vi "Periodic Tasks.vi"(8 "error in":errorcluster) -> ()   [LabVIEW 2011]
doc: "This VI runs in parallel to other tasks. It can contain as many user-defined periodic loops as you need. These can carry out PID or other sorts of timed response."
uses:
  <vilib>/Rock Robotics/WPI/DriverStation/WPI_DriverStationRobotMode.ctl
  <vilib>/Rock Robotics/SystemInterfaces/Utilities/FPGA_UtilitiesLED State.ctl
  <vilib>/Rock Robotics/SystemInterfaces/Utilities/FPGA_UtilitiesLED Source.ctl
  Robot Global Data.vi
  <vilib>/Rock Robotics/WPI/Solenoid/Deprecated/WPI_SolenoidSetBool.vi
  <vilib>/Rock Robotics/WPI/Compressor/WPI_CompressorGetSetRefNum.vi
  <vilib>/addons/control/pid/NI_PID_pid.lvlib
  <vilib>/addons/control/pid/pid.llb/PID (DBL).vi
panel:
  out "Turret Joystick":dbl(slide) scale=-1.0..1.0
  out "PID Output":dbl(slide) scale=-1.0..1.0
  out "Target Pot":dbl(slide) scale=2.0..3.5
  in  "Min Turret Output":dbl
  # "!!!DISABLED!!!"
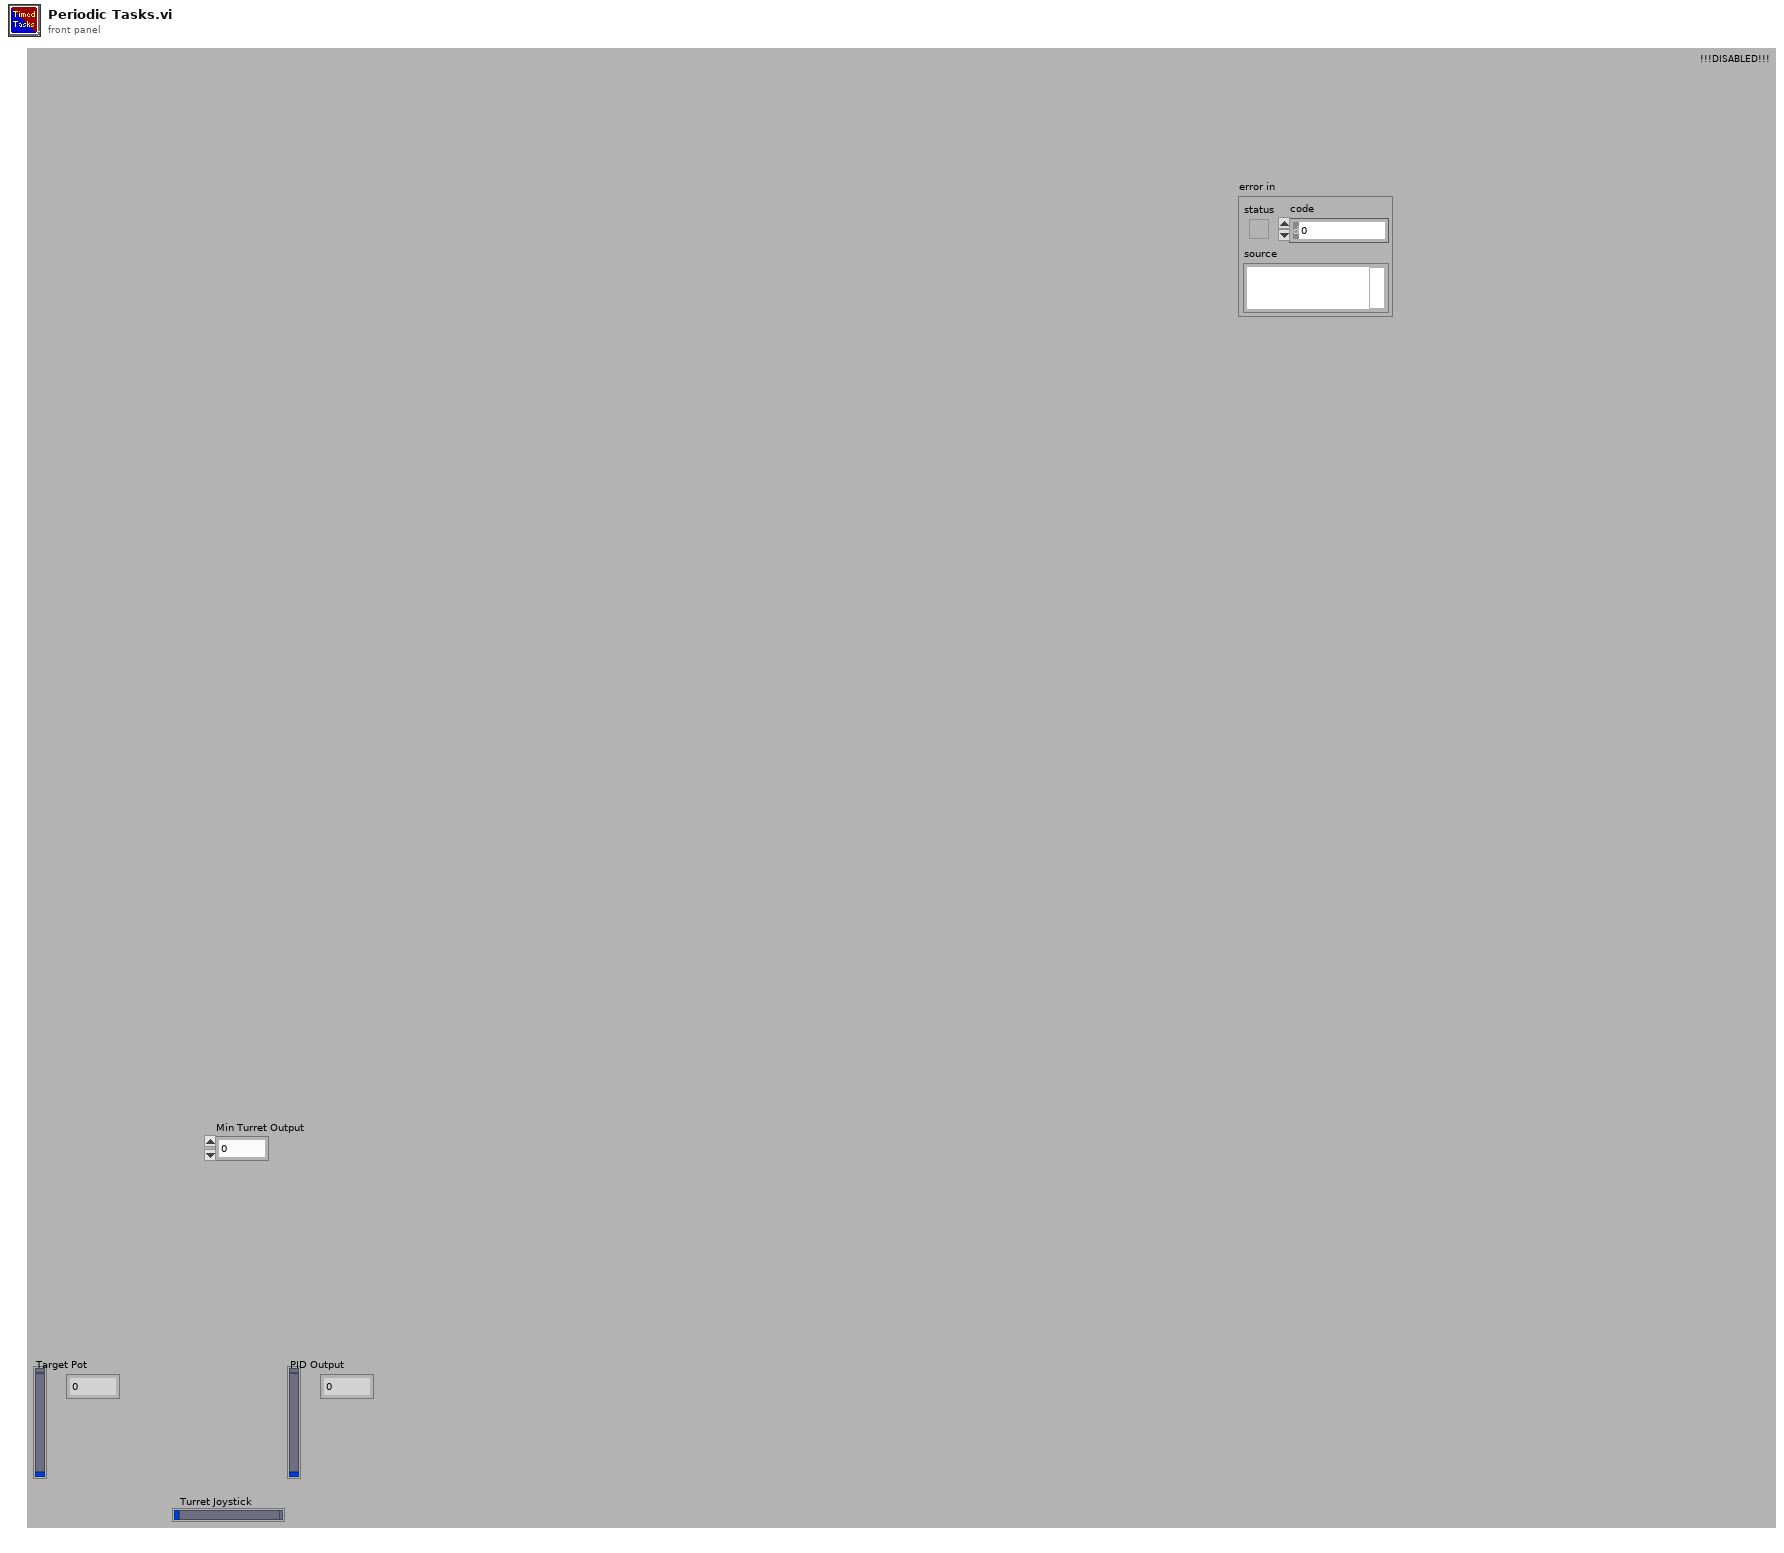
[diagram p1: front panel]
types:
  T1 = typedef "WPI_DriverStationRobotMode.ctl" = enum16{"Autonomous Disabled", "Autonomous Enabled", "Teleop Disabled", "Teleop Enabled", "Timeout", "Finish"}
  T2 = cluster{"proportional gain (Kc)":dbl, "integral time (Ti, min)":dbl, "derivative time (Td, min)":dbl}
  T3 = typedef "WPI_AnalogChannelDevRef.ctl" = cluster{"DevStatus":errorcluster, "Analog Module":T4, "Analog Channel":T5}
  T4 = typedef "FPGA_TypedefAnalogModule.ctl" = enum16{"Analog Module 1", "Analog Module 2"}
  T5 = typedef "FPGA_AIChannel.ctl" = enum8{"AI 1", "AI 2", "AI 3", "AI 4", "AI 5", "AI 6", "AI 7", "AI 8", "Invalid"}
  T6 = typedef "WPI_MotorControlDeviceRef.ctl" = cluster{"DeviceStatus":errorcluster, "Type":enum16{"PWM", "CAN"}, "PWM":cluster{"Digital Module":T7, "PWM Channel":T8, "DeadBand":T9}, "CAN":cluster{"Device Number":u8, "Control Mode":T10, "Semaphore":T11, "Max Vout":dbl}, "Invert":bool, "TransformRef":T12, "InvTransformRef":T12}
  T7 = typedef "FPGA_TypedefDigitalModule.ctl" = enum16{"Digital Module 1", "Digital Module 2"}
  T8 = typedef "FPGA_DIOPWMChannel.ctl" = enum8{"PWM 1", "PWM 2", "PWM 3", "PWM 4", "PWM 5", "PWM 6", "PWM 7", "PWM 8", "PWM 9", "PWM 10", "Invalid"}
  T9 = typedef "WPI_PWMDeadband.ctl" = cluster{"Name":string, "maxPositivePwm":i32, "minPositivePwm":i32, "centerPwm":i32, "maxNegativePwm":i32, "minNegativePwm":i32, "angularRange":u16}
  T10 = typedef "WPI_CANJaguar_ControlMode.ctl" = enum8{"Percent VBus", "Current", "Speed", "Position", "Voltage"}
  T11 = typedef "Semaphore RefNum" = refnum<k1>
  T12 = typedef "WPI_PWMTransform_ConPane.ctl" = refnum<vi>
  T13 = cluster{"axis 1 (x)":dbl, "axis 2 (y)":dbl, "axis 3 (throttle)":dbl, "axis 4":dbl, "axis 5":dbl, "axis 6":dbl}
  T14 = typedef "WPI_JoystickButtonState.ctl" = cluster{"Button 1":bool, "Button 2":bool, "Button 3":bool, "Button 4":bool, "Button 5":bool, "Button 6":bool, "Button 7":bool, "Button 8":bool, "Button 9":bool, "Button 10":bool, "Button 11":bool, "Button 12":bool}
  T15 = typedef "UDP Dashboard Packet TypeDef.ctl" = cluster{"Distance":dbl, "Shooter Control":cluster{"Manual Enabled":bool, "Manual Distance":dbl, "Power Constant":dbl, "RPM Constant":dbl, "Layup Distance":dbl, "RPM Range":cluster{"Max Percentage":dbl, "Min Percentage":dbl}, "Dt In":dbl}, "Tracking Setpoint":dbl, "Shooter PID gains":cluster{"proportional gain (Kc)":dbl, "integral time (Ti, min)":dbl, "derivative time (Td, min)":dbl}, "Tracking PID gains":cluster{"proportional gain (Kc)":dbl, "integral time (Ti, min)":dbl, "derivative time (Td, min)":dbl}, "Shooter PID gains 2":cluster{"proportional gain (Kc)":dbl, "integral time (Ti, min)":dbl, "derivative time (Td, min)":dbl}, "Tracking Tolerance":dbl, "Tracking Limit":dbl, "Autonomous Ball Collection / Shoot Period":dbl}
  T16 = cluster{"Target Pot":dbl, "Motor Output":dbl, "Current Voltage":dbl}
  T17 = typedef "WPI_CompressorDevRef.ctl" = cluster{"DevStatus":errorcluster, "DigitalInputDevRef":T18, "RelayDevRef":T20}
  T18 = typedef "WPI_DigitalInputDevRef.ctl" = cluster{"DevStatus":errorcluster, "DIO Channel":T19, "Digital Module":T7}
  T19 = typedef "FPGA_DIOChannel.ctl" = enum8{"DIO 1", "DIO 2", "DIO 3", "DIO 4", "DIO 5", "DIO 6", "DIO 7", "DIO 8", "DIO 9", "DIO 10", "DIO 11", "DIO 12", "DIO 13", "DIO 14", "Invalid"}
  T20 = typedef "WPI_RelayDevRef.ctl" = cluster{"DevStatus":errorcluster, "Relay Channel":T21, "Digital Module":T7, "Relay Direction":T22}
  T21 = typedef "FPGA_DIORelayChannel.ctl" = enum8{"Relay 1", "Relay 2", "Relay 3", "Relay 4", "Relay 5", "Relay 6", "Relay 7", "Relay 8", "Invalid"}
  T22 = typedef "WPI_RelayDirection.ctl" = enum16{"Both directions", "Forward only", "Reverse only"}
  T23 = typedef "WPI_SolenoidDevRef.ctl" = cluster{"DevStatus":errorcluster, "Solenoid Module":T24, "Forward Solenoid Channel":T25, "Reverse Solenoid Channel":T25}
  T24 = typedef "FPGA_TypedefSolenoidModule.ctl" = enum16{"Solenoid Module 1", "Solenoid Module 2"}
  T25 = typedef "WPI_SolenoidChannel.ctl" = enum8{"Solenoid 1", "Solenoid 2", "Solenoid 3", "Solenoid 4", "Solenoid 5", "Solenoid 6", "Solenoid 7", "Solenoid 8", "Invalid"}
  T26 = typedef "WPI_GyroDevRef.ctl" = cluster{"DevStatus":errorcluster, "Analog Module":T4, "Analog Channel":T5, "Offset":dbl, "Gain (VoltsPerDegree/Second)":dbl}
  T27 = cluster{"Gear Shifter":bool, "Tipper":bool, "Tipper Lock":bool, "Stabilizer":bool}
  T28 = cluster{"Shooter Warmup":bool, "Shooter Allow Fire":bool}
  T29 = cluster{"Front Roller":bool, "Back Roller":bool, "Lower Mag":bool, "Upper Mag":bool, "Front Enter":bool, "Rear Enter":bool}
  T30 = cluster{"Current State":u32, "Reading State":u32, "Number of Balls":u32, "State":enum16{"Load Balls", "Shoot", "Wait"}}
  T31 = typedef "FPGA_UtilitiesLED State.ctl" = enum16{"Off", "On", "Toggle"}
  T32 = typedef "FPGA_UtilitiesLED Source.ctl" = enum16{"User LED", "FPGA LED"}
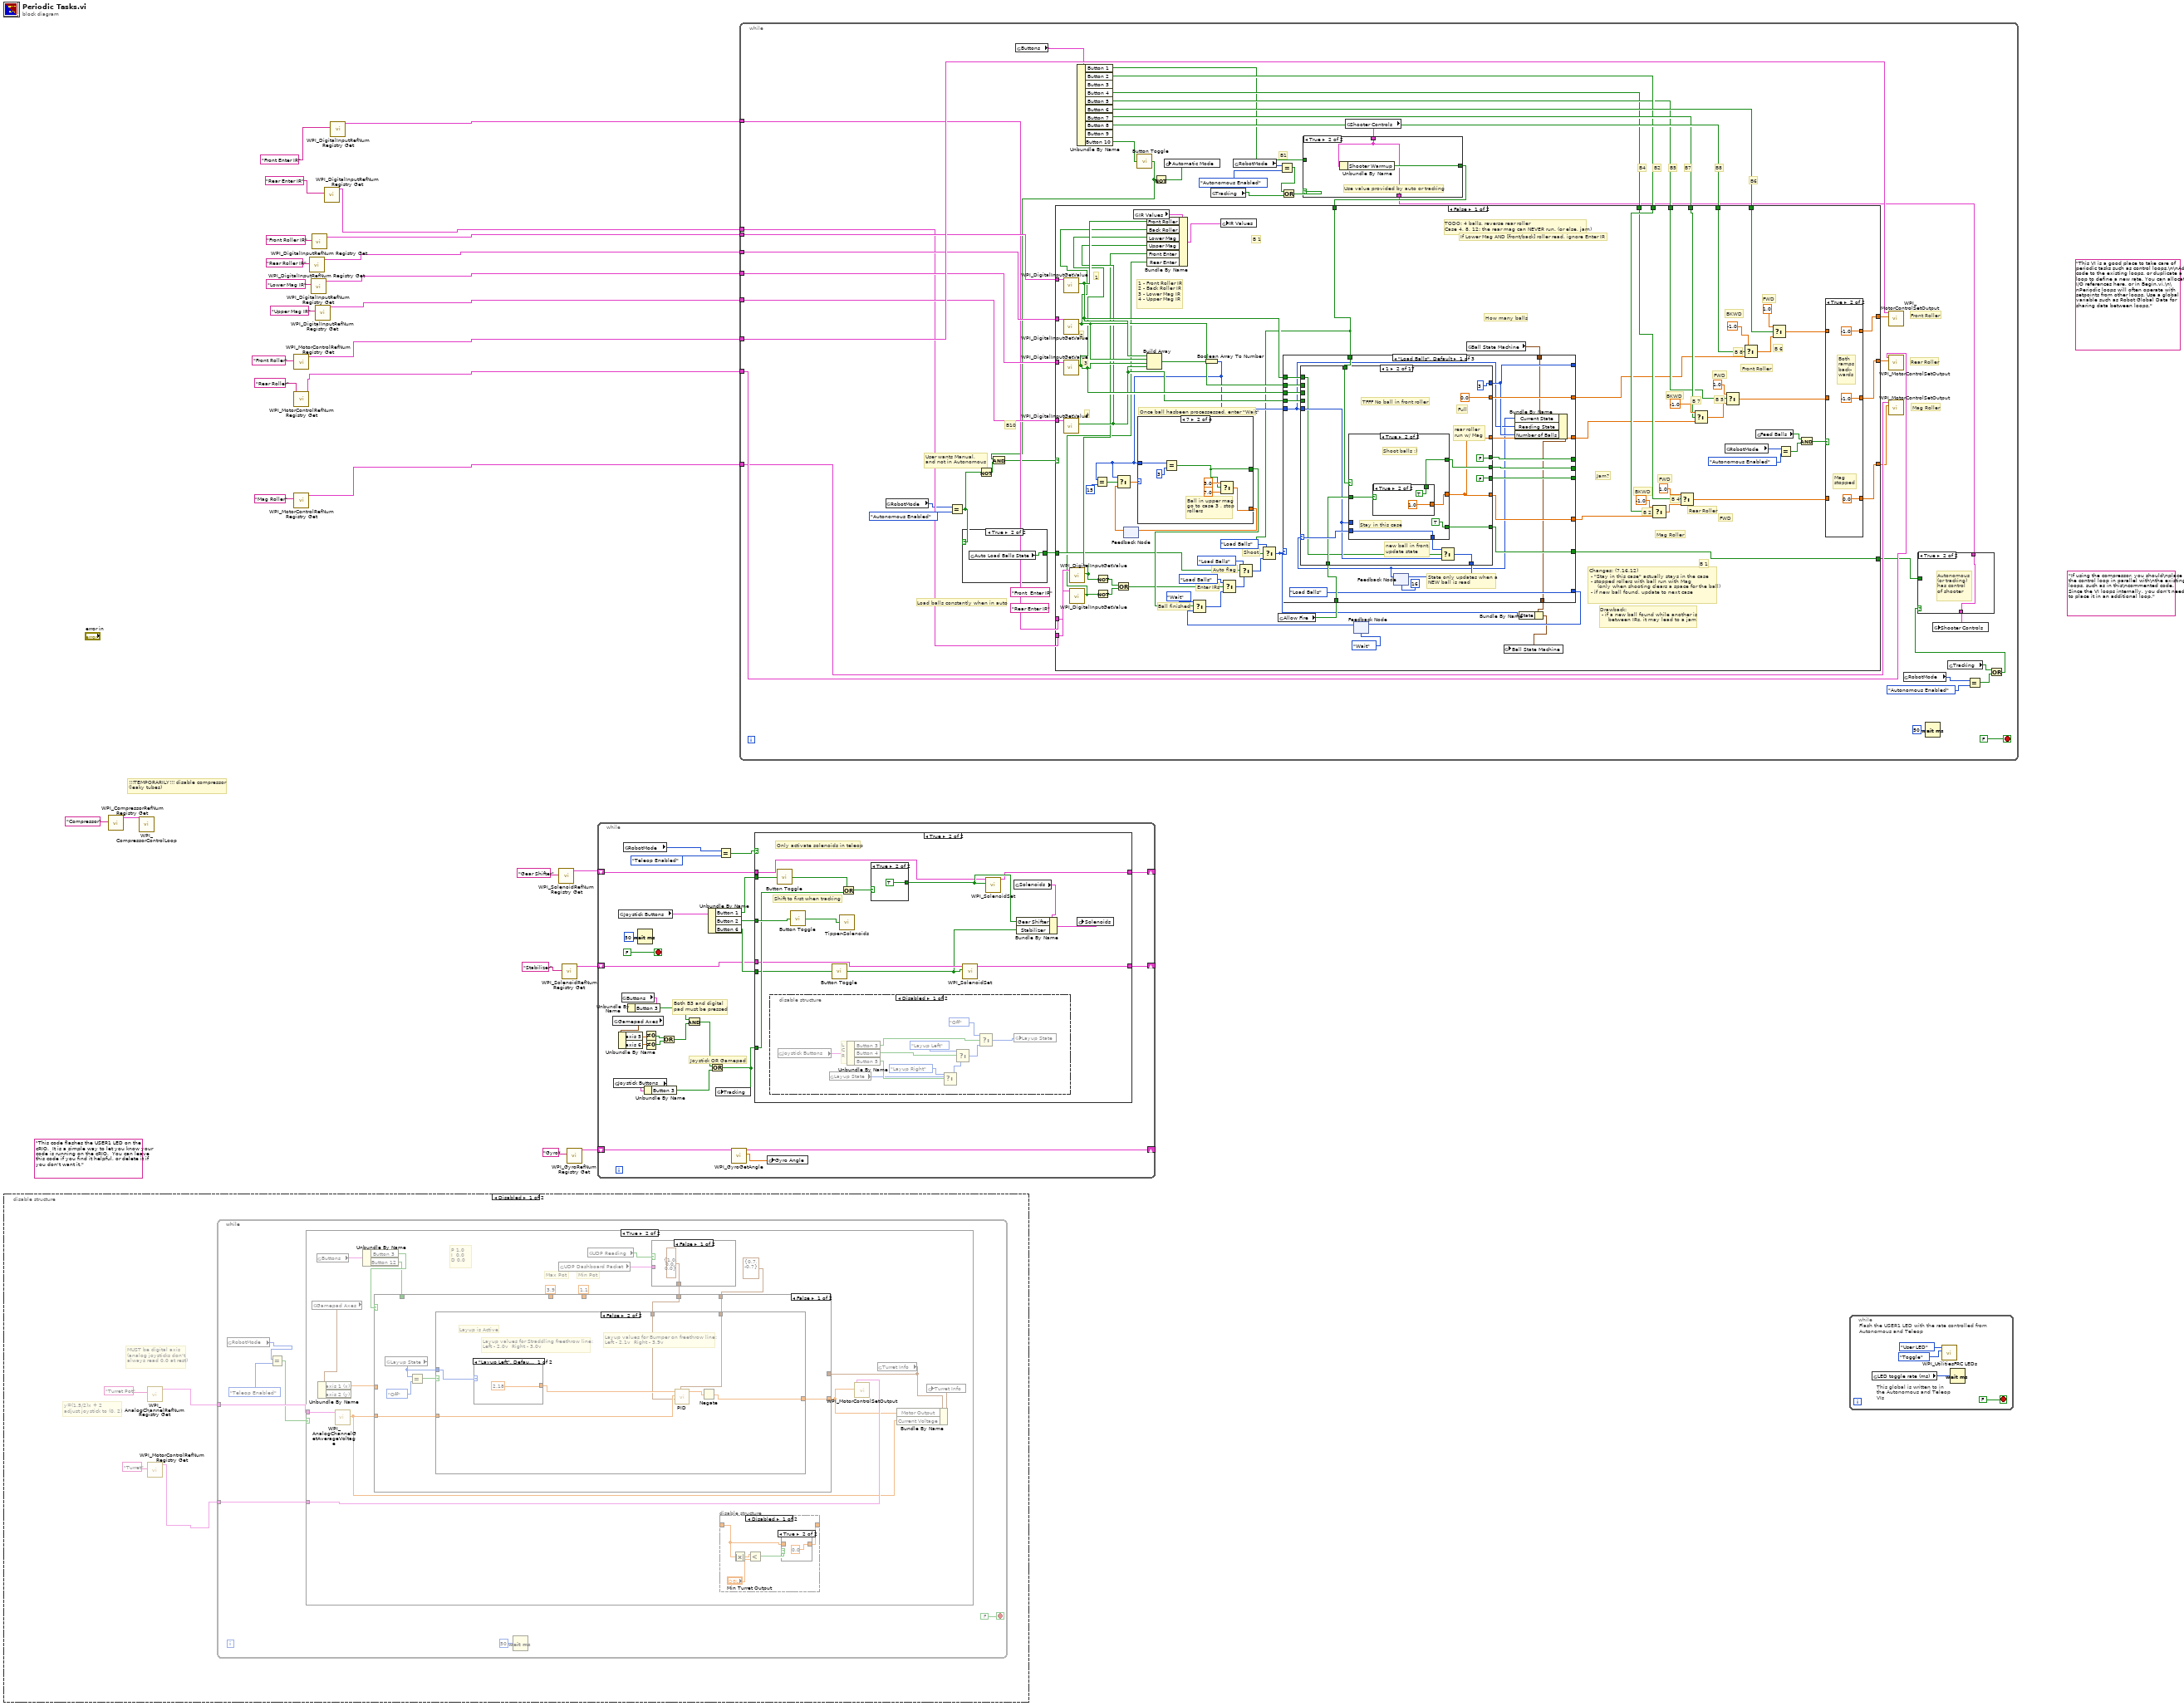
[diagram p0: block diagram]
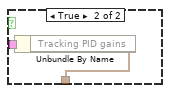
[diagram p3: hidden frame]
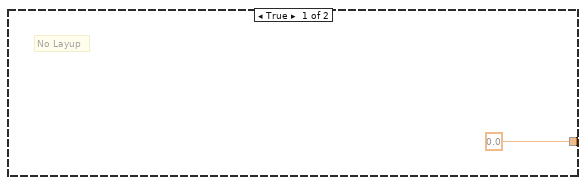
[diagram p4: hidden frame]
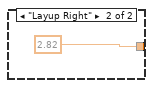
[diagram p5: hidden frame]
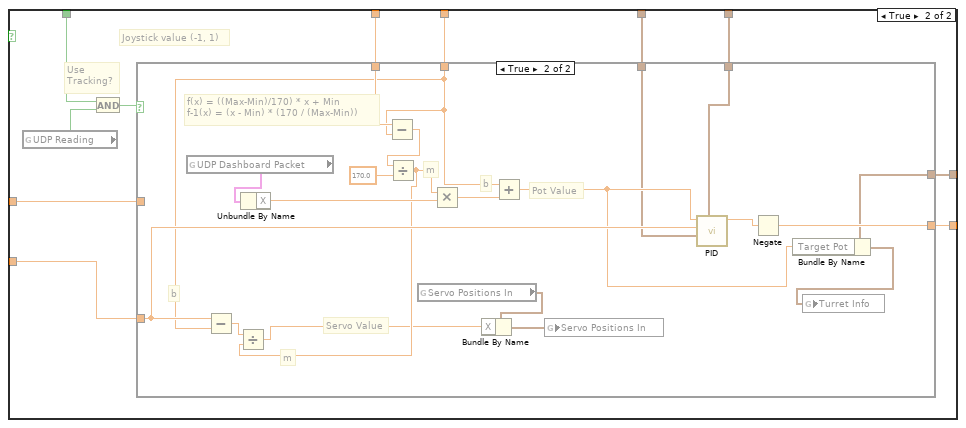
[diagram p6: hidden frame]
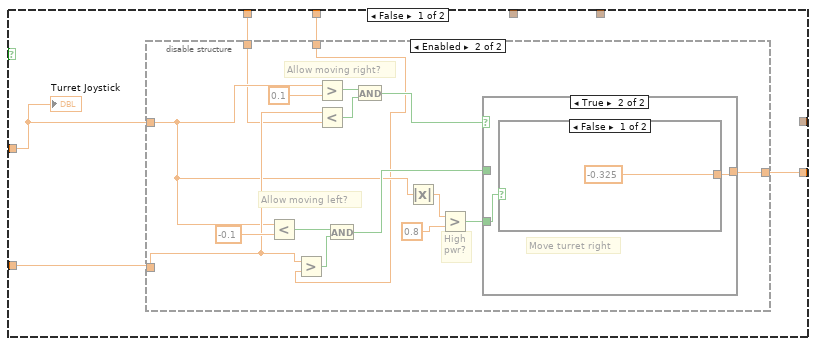
[diagram p7: hidden frame]
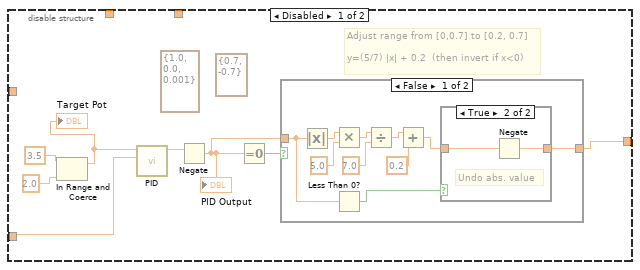
[diagram p8: hidden frame]
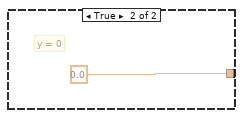
[diagram p10: hidden frame]
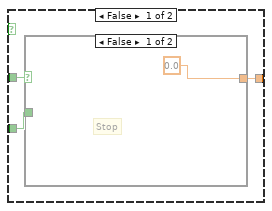
[diagram p11: hidden frame]
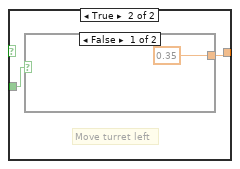
[diagram p12: hidden frame]
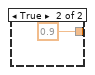
[diagram p13: hidden frame]
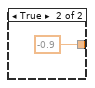
[diagram p14: hidden frame]
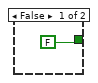
[diagram p20: hidden frame]
diagram:
  (unwired) "If using the compressor, you should\nplace the control loop in parallel with\nthe existing loops, such as in this\ncommented code. Since the VI loops internally, you don't need to place it in an additional loop."
  (unwired) "This code flashes the USER1 LED on the cRIO.  It is a simple way to let you know your code is running on the cRIO.  You can leave this code if you find it helpful, or delete it if you don't want it."
  (unwired) "This VI is a good place to take care of periodic tasks such as control loops.\n\nAdd code to the existing loops, or duplicate a loop to define a new rate. You can allocate I/O references here, or in Begin.vi.\n\nPeriodic loops will often operate with setpoints from other loops. Use a global variable such as Robot Global Data for sharing data between loops."
  # "!!!TEMPORARILY!!! disable compressor\n(leaky tubes)"
  n1 = disable-structure shown="Disabled" {
    frame Disabled {
      # "MUST be digital axis\n(analog joysticks don't\nalways read 0.0 at rest)"
      # "y=(1.5/2)x + 2\nadjust joystick to (0, 2)"
      n2 = call <vilib>:"WPI_AnalogChannelRefNum Registry Get.vi"("refnum name"="Turret Pot") -> ("AIDeviceRef"=w28:T3)  [unwired: 9 in, 1 out]
      n3 = call <vilib>:"WPI_MotorControlRefNum Registry Get.vi"("refnum name"="Turret") -> ("MotorControlDevRef"=w27:T6)  [unwired: 9 in, 1 out]
      n4 = while {
        tunnel: w27 -> [w36]
        tunnel: w28 -> [w34]
        stop <- FALSE stop-if-true
        n5 = global read "Robot Global Data.vi" "RobotMode"() -> (w33:T1)
        n6 = Equal?(x=w33, y=WPI_DriverStationRobotMode."Teleop Enabled" ("Robot Mode")) -> (x = y?=w31:bool)
        n7 = case shown="True" w31 {
          tunnel: w36 -> [_ w50]
          tunnel: w34 -> [_ w42]
          frame False {
          }
          frame True {
            # "Min Pot"
            # "Max Pot"
            # "P 1.0\nI  0.0\nD 0.0"
            n8 = global read "Robot Global Data.vi" "Gamepad Axes"() -> (w53:T13)
            n9 = global read "Robot Global Data.vi" "Buttons"() -> (w54:T14)
            n10 = Unbundle By Name(w53) -> ("axis 1 (x)"=w52:dbl)  [unwired: 1 out]
            n11 = call <vilib>:"WPI_AnalogChannelGetAverageVoltage.vi"("AIDeviceRef"=w42) -> ("Voltage"=w44:dbl)  [unwired: 8 in, 2 out]
            n12 = Unbundle By Name(w54) -> ("Button 3"=w51:bool, "Button 12"=w49:bool)
            n13 = global read "Robot Global Data.vi" "UDP Dashboard Packet"() -> (w39:T15)
            n14 = global read "Robot Global Data.vi" "UDP Reading"() -> (w40:bool)
            n15 = case shown="False" w40 {
              tunnel: [T2 {"proportional gain (Kc)"=1.0, "integral time (Ti, min)"=0.0, "derivative time (Td, min)"=0.0} ("PID gains") w56] -> w41
              tunnel: w39 -> [_ w57]
              frame False {
              }
              frame True {
                n16 = Unbundle By Name(w57) -> ("Tracking PID gains"=w56:T2)
              }
            }
            n17 = disable-structure shown="Disabled" {
              disable-tunnel: _ -> [w162 _]
              disable-tunnel: [w161 _] -> _
              frame Disabled {
                n18 = Absolute Value(x=w162) -> (abs(x)=w165:dbl)
                n19 = Less?(x=w165, y="Min Turret Output") -> (x < y?=w163:bool)
                n20 = case shown="True" w163 {
                  tunnel: [w166 0.0] -> w161
                  tunnel: w162 -> [w166 _]
                  frame False {
                  }
                  frame True {
                  }
                }
              }
              frame Enabled {
              }
            }
            n21 = global read "Robot Global Data.vi" "Turret Info"() -> (w43:T16)
            n22 = case shown="False" w51 {
              tunnel: w52 -> [_ w83]
              tunnel: w44 -> [w63 w85]
              tunnel: [w64 w84] -> w45
              tunnel: w49 -> [_ w81]
              tunnel: 3.9 ("y") -> [_ w79]
              tunnel: 1.1 ("y") -> [_ w78]
              tunnel: w43 -> [_ w77]
              tunnel: w41 -> [w58 w76]
              tunnel: cluster{"output high":dbl, "output low":dbl} {"output high"=0.7, "output low"=-0.7} ("output range") -> [w59 w75]
              frame False {
                n23 = global read "Robot Global Data.vi" "Layup State"() -> (w60:enum16{"Layup Left", "Layup Right", "Off"})
                n24 = Equal?(x=w60, y=enum16{"Layup Left", "Layup Right", "Off"}."Off") -> (x = y?=w62:bool)
                n25 = case shown="False" w62 {
                  tunnel: [0.0 w71] -> w64
                  tunnel: w63 -> [_ w70]
                  tunnel: w60 -> [_ w69]
                  tunnel: w59 -> [_ w67]
                  tunnel: w58 -> [_ w66]
                  frame True {
                    # "No Layup"
                  }
                  frame False {
                    # "Layup values for Bumper on freethrow line:\nLeft - 2.1v  Right - 3.9v"
                    # "Layup values for Straddling freethrow line:\nLeft - 2.0v  Right - 3.0v"
                    # "Layup is Active"
                    n26 = case shown="\"Layup Left\", Default" w69 {
                      tunnel: [2.18 ("y") 2.82 ("y")] -> w68
                      frame "Layup Left", Default {
                      }
                      frame "Layup Right" {
                      }
                    }
                    n27 = call-poly <vilib>:"PID.vi"("output range"=w67, "PID gains"=w66, "process variable"=w70, "setpoint"=w68) -> ("output"=w72:dbl)  [unwired: 6 in, 1 out]
                    n28 = Negate(x=w72) -> (-x=w71:dbl)
                  }
                }
              }
              frame True {
                # "Use \nTracking?"
                # "Joystick value (-1, 1)"
                n29 = global read "Robot Global Data.vi" "UDP Reading"() -> (w82:bool)
                n30 = And(x=w81, y=w82) -> (x .and. y?=w80:bool)
                n31 = case shown="True" w80 {
                  tunnel: w85 -> [w90 w148]
                  tunnel: [w89 w154] -> w84
                  tunnel: w83 -> [w88 _]
                  tunnel: w79 -> [w87 w159]
                  tunnel: w78 -> [w86 w147]
                  tunnel: w77 -> [_ w151]
                  tunnel: w76 -> [_ w142]
                  tunnel: w75 -> [_ w141]
                  frame False {
                    n32 = disable-structure shown="Enabled" {
                      disable-tunnel: w90 -> [w96 w119]
                      disable-tunnel: [w91 w128] -> w89
                      disable-tunnel: w88 -> [_ w116]
                      disable-tunnel: w87 -> [_ w114]
                      disable-tunnel: w86 -> [_ w113]
                      frame Disabled {
                        (unwired) T2 {"proportional gain (Kc)"=1.0, "integral time (Ti, min)"=0.0, "derivative time (Td, min)"=0.001} ("PID gains")
                        (unwired) cluster{"output high":dbl, "output low":dbl} {"output high"=0.7, "output low"=-0.7} ("output range")
                        # "Adjust range from [0,0.7] to [0.2, 0.7]\n\ny=(5/7) |x| + 0.2  (then invert if x<0)"
                        n33 = In Range and Coerce(upper limit=3.5, lower limit=2.0) -> (coerced(x)=w95:dbl)  [unwired: 1 in, 1 out]
                        "Target Pot" <- w95
                        n34 = call-poly <vilib>:"PID.vi"("process variable"=w96, "setpoint"=w95) -> ("output"=w94:dbl)  [unwired: 8 in, 1 out]
                        n35 = Negate(x=w94) -> (-x=w92:dbl)
                        "PID Output" <- w92
                        n36 = Equal To 0?(x=w92) -> (x = 0?=w93:bool)
                        n37 = case shown="False" w93 {
                          tunnel: w92 -> [w102 _]
                          tunnel: [w99 0.0] -> w91
                          frame False {
                            n38 = Absolute Value(x=w102) -> (abs(x)=w108:dbl)
                            n39 = Multiply(x=w108, y=5.0) -> (x*y=w107:dbl)
                            n40 = Less Than 0?(x=w102) -> (x < 0?=w101:bool)
                            n41 = Divide(x=w107, y=7.0) -> (x/y=w105:dbl)
                            n42 = Add(x=w105, y=0.2) -> (x+y=w100:dbl)
                            n43 = case shown="True" w101 {
                              tunnel: w100 -> [w109 w111]
                              tunnel: [w109 w110] -> w99
                              frame False {
                              }
                              frame True {
                                # "Undo abs. value"
                                n44 = Negate(x=w111) -> (-x=w110:dbl)
                              }
                            }
                          }
                          frame True {
                            # "y = 0"
                          }
                        }
                      }
                      frame Enabled {
                        # "High\npwr?"
                        # "Allow moving left?"
                        # "Allow moving right?"
                        n45 = Less?(x=w116, y=-0.1) -> (x < y?=w127:bool)
                        n46 = Greater?(x=w119, y=w113) -> (0:w126:bool)
                        n47 = Greater?(x=w116, y=0.1) -> (0:w123:bool)
                        n48 = Less?(x=w119, y=w114) -> (x < y?=w122:bool)
                        n49 = And(x=w127, y=w126) -> (x .and. y?=w125:bool)
                        n50 = And(x=w123, y=w122) -> (x .and. y?=w124:bool)
                        n51 = Absolute Value(x=w116) -> (abs(x)=w117:dbl)
                        n52 = Greater?(x=w117, y=0.8 ("upper limit")) -> (0:w115:bool)
                        n53 = case shown="True" w124 {
                          tunnel: [w130 w138] -> w128
                          tunnel: w125 -> [w131 _]
                          tunnel: w115 -> [w129 w137]
                          frame False {
                            n54 = case shown="False" w131 {
                              tunnel: [0.0 w134] -> w130
                              tunnel: w129 -> [_ w133]
                              frame False {
                                # "Stop"
                              }
                              frame True {
                                # "Move turret left"
                                n55 = case shown="False" w133 {
                                tunnel: [0.35 0.9] -> w134
                                frame False {
                                }
                                frame True {
                                }
                                }
                              }
                            }
                          }
                          frame True {
                            # "Move turret right"
                            n56 = case shown="False" w137 {
                              tunnel: [-0.325 -0.9] -> w138
                              frame False {
                              }
                              frame True {
                              }
                            }
                          }
                        }
                      }
                    }
                    "Turret Joystick" <- w88
                  }
                  frame True {
                    # "Servo Value"
                    # "Pot Value"
                    # "f(x) = ((Max-Min)/170) * x + Min\nf-1(x) = (x - Min) * (170 / (Max-Min))"
                    # "m"
                    # "b"
                    # "b"
                    # "m"
                    n57 = global read "Robot Global Data.vi" "UDP Dashboard Packet"() -> (w160:T15)
                    n58 = Subtract(x=w148, y=w147) -> (x-y=w146:dbl)
                    n59 = Unbundle By Name(w160) -> ("X"=w155:dbl)
                    n60 = Subtract(x=w159, y=w147) -> (x-y=w158:dbl)
                    n61 = Divide(x=w158, y=170.0) -> (x/y=w145:dbl)
                    n62 = Divide(x=w146, y=w145) -> (x/y=w144:dbl)
                    n63 = global read "Robot Global Data.vi" "Servo Positions In"() -> (w149:cluster{"X":dbl, "Y":dbl})
                    n64 = Multiply(x=w145, y=w155) -> (x*y=w156:dbl)
                    n65 = Bundle By Name(cluster=w149, "X"=w144) -> (w150:cluster{"X":dbl, "Y":dbl})
                    n66 = Add(x=w147, y=w156) -> (x+y=w143:dbl)
                    n67 = global write "Robot Global Data.vi" "Servo Positions In"(w150) -> ()
                    n68 = call-poly <vilib>:"PID.vi"("output range"=w141, "PID gains"=w142, "process variable"=w148, "setpoint"=w143) -> ("output"=w153:dbl)  [unwired: 6 in, 1 out]
                    n69 = Negate(x=w153) -> (-x=w154:dbl)
                    n70 = Bundle By Name(cluster=w151, "Target Pot"=w143) -> (w152:T16)
                    n71 = global write "Robot Global Data.vi" "Turret Info"(w152) -> ()
                  }
                }
              }
            }
            n72 = call <vilib>:"WPI_MotorControlSetOutput.vi"("Output"=w45, "MotorControlDevRef"=w50) -> ()  [unwired: 8 in, 2 out]
            n73 = Bundle By Name(cluster=w43, "Motor Output"=w45, "Current Voltage"=w44) -> (w46:T16)
            n74 = global write "Robot Global Data.vi" "Turret Info"(w46) -> ()
          }
        }
        n75 = Wait (ms)(milliseconds to wait=u32 50) -> ()  [unwired: 1 out]
      }
    }
    frame Enabled {
    }
  }
  n76 = call <vilib>:"WPI_CompressorRefNum Registry Get.vi"("refnum name"="Compressor") -> ("CompressorDevRef"=w23:T17)  [unwired: 9 in, 1 out]
  n77 = call <vilib>:"WPI_CompressorControlLoop.vi"("CompressorDevRef"=w23) -> ()  [unwired: 11 in]
  n78 = call <vilib>:"WPI_MotorControlRefNum Registry Get.vi"("refnum name"="Front Roller") -> ("MotorControlDevRef"=w8:T6)  [unwired: 9 in, 1 out]
  n79 = call <vilib>:"WPI_MotorControlRefNum Registry Get.vi"("refnum name"="Rear Roller") -> ("MotorControlDevRef"=w7:T6)  [unwired: 9 in, 1 out]
  n80 = call <vilib>:"WPI_MotorControlRefNum Registry Get.vi"("refnum name"="Mag Roller") -> ("MotorControlDevRef"=w6:T6)  [unwired: 9 in, 1 out]
  n81 = call <vilib>:"WPI_DigitalInputRefNum Registry Get.vi"("refnum name"="Rear Roller IR") -> ("DigitalInputDevRef"=w11:T18)  [unwired: 9 in, 1 out]
  n82 = call <vilib>:"WPI_DigitalInputRefNum Registry Get.vi"("refnum name"="Lower Mag IR") -> ("DigitalInputDevRef"=w10:T18)  [unwired: 9 in, 1 out]
  n83 = call <vilib>:"WPI_DigitalInputRefNum Registry Get.vi"("refnum name"="Front Roller IR") -> ("DigitalInputDevRef"=w12:T18)  [unwired: 9 in, 1 out]
  n84 = call <vilib>:"WPI_DigitalInputRefNum Registry Get.vi"("refnum name"="Upper Mag IR") -> ("DigitalInputDevRef"=w9:T18)  [unwired: 9 in, 1 out]
  n85 = call <vilib>:"WPI_DigitalInputRefNum Registry Get.vi"("refnum name"="Rear Enter IR") -> ("DigitalInputDevRef"=w13:T18)  [unwired: 9 in, 1 out]
  n86 = call <vilib>:"WPI_DigitalInputRefNum Registry Get.vi"("refnum name"="Front Enter IR") -> ("DigitalInputDevRef"=w14:T18)  [unwired: 9 in, 1 out]
  n87 = call <vilib>:"WPI_SolenoidRefNum Registry Get.vi"("refnum name"="Gear Shifter") -> ("SolenoidDevRef"=w5:T23)  [unwired: 9 in, 1 out]
  n88 = call <vilib>:"WPI_SolenoidRefNum Registry Get.vi"("refnum name"="Stabilizer") -> ("SolenoidDevRef"=w2:T23)  [unwired: 9 in, 1 out]
  n89 = call <vilib>:"WPI_GyroRefNum Registry Get.vi"("refnum name"="Gyro") -> ("GyroDevRef"=w3:T26)  [unwired: 9 in, 1 out]
  n90 = while {
    shift-right: [w188] -> _
    shift-left: w5 -> [w190]
    shift-right: [w183] -> _
    shift-left: w3 -> [w185]
    shift-right: [w168] -> _
    shift-left: w2 -> [w169]
    stop <- FALSE stop-if-true
    # "Joystick OR Gamepad"
    # "Both B3 and digital\npad must be pressed"
    n91 = global read "Robot Global Data.vi" "Gamepad Axes"() -> (w181:T13)
    n92 = global read "Robot Global Data.vi" "Joystick Buttons"() -> (w174:T14)
    n93 = Unbundle By Name(w181) -> ("axis 5"=w180:dbl, "axis 6"=w179:dbl)
    n94 = global read "Robot Global Data.vi" "Joystick Buttons"() -> (w195:T14)
    n95 = global read "Robot Global Data.vi" "Buttons"() -> (w182:T14)
    n96 = global read "Robot Global Data.vi" "RobotMode"() -> (w194:T1)
    n97 = Unbundle By Name(w182) -> ("Button 3"=w176:bool)
    n98 = Wait (ms)(milliseconds to wait=u32 50) -> ()  [unwired: 1 out]
    n99 = Not Equal To 0?(x=w180) -> (x != 0?=w178:bool)
    n100 = Not Equal To 0?(x=w179) -> (x != 0?=w177:bool)
    n101 = Unbundle By Name(w174) -> ("Button 3"=w171:bool)
    n102 = Or(x=w178, y=w177) -> (x .or. y?=w175:bool)
    n103 = And(x=w176, y=w175) -> (x .and. y?=w172:bool)
    n104 = Unbundle By Name(w195) -> ("Button 1"=w191:bool, "Button 2"=w186:bool, "Button 6"=w170:bool)
    n105 = Or(x=w172, y=w171) -> (x .or. y?=w173:bool)
    n106 = global write "Robot Global Data.vi" "Tracking"(w173) -> ()
    n107 = Equal?(x=w194, y=WPI_DriverStationRobotMode."Teleop Enabled" ("Robot Mode")) -> (x = y?=w192:bool)
    n108 = call <vilib>:"WPI_GyroGetAngle.vi"("GyroDevRef"=w185) -> ("Angle"=w184:dbl, "GyroDevRef"=w183:T26)  [unwired: 7 in, 2 out]
    n109 = case shown="True" w192 {
      tunnel: w191 -> [_ w209]
      tunnel: w190 -> [w197 w208]
      tunnel: [w197 w207] -> w188
      tunnel: w186 -> [_ w206]
      tunnel: w173 -> [_ w202]
      tunnel: w170 -> [_ w201]
      tunnel: w169 -> [w196 w200]
      tunnel: [w196 w199] -> w168
      frame False {
        # "Do NOTHING\nwhen not in Teleop"
      }
      frame True {
        # "Shift to first when tracking"
        # "Only activate solenoids in teleop"
        n110 = disable-structure shown="Disabled" {
          frame Disabled {
            # "L\nC\nR"
            n111 = global read "Robot Global Data.vi" "Joystick Buttons"() -> (w223:T14)
            n112 = global read "Robot Global Data.vi" "Layup State"() -> (w221:enum16{"Layup Left", "Layup Right", "Off"})
            n113 = Unbundle By Name(w223) -> ("Button 3"=w218:bool, "Button 4"=w220:bool, "Button 5"=w222:bool)
            n114 = Select(t=enum16{"Layup Left", "Layup Right", "Off"}."Layup Right" ("Layup State"), s=w222, f=w221) -> (s? t:f=w219:enum16{"Layup Left", "Layup Right", "Off"})
            n115 = Select(t=enum16{"Layup Left", "Layup Right", "Off"}."Layup Left" ("Layup State"), s=w220, f=w219) -> (s? t:f=w217:enum16{"Layup Left", "Layup Right", "Off"})
            n116 = Select(t=enum16{"Layup Left", "Layup Right", "Off"}."Off" ("Layup State"), s=w218, f=w217) -> (s? t:f=w213:enum16{"Layup Left", "Layup Right", "Off"})
            n117 = global write "Robot Global Data.vi" "Layup State"(w213) -> ()
          }
          frame Enabled {
          }
        }
        n118 = call "Button Toggle.vi"("Button Input"=w209) -> ("Toggled Output"=w204:bool)
        n119 = call "Button Toggle.vi"("Button Input"=w206) -> ("Toggled Output"=w205:bool)
        n120 = call "Button Toggle.vi"("Button Input"=w201) -> ("Toggled Output"=w198:bool)
        n121 = call "Tipper-Solenoids.vi"("Deploy Tipper"=w205) -> ()  [unwired: 1 out]
        n122 = Or(x=w204, y=w202) -> (x .or. y?=w203:bool)
        n123 = case shown="True" w203 {
          tunnel: [FALSE TRUE] -> w211
          frame False {
          }
          frame True {
          }
        }
        n124 = call-poly <vilib>:"WPI_SolenoidSet.vi"("Value"=w198, "SolenoidDevRef"=w200) -> ("SolenoidDevRef"=w199:T23)  [unwired: 8 in, 1 out]
        n125 = call-poly <vilib>:"WPI_SolenoidSet.vi"("Value"=w211, "SolenoidDevRef"=w208) -> ("SolenoidDevRef"=w207:T23)  [unwired: 8 in, 1 out]
        n126 = global read "Robot Global Data.vi" "Solenoids"() -> (w210:T27)
        n127 = Bundle By Name(cluster=w210, "Gear Shifter"=w211, "Stabilizer"=w198) -> (w212:T27)
        n128 = global write "Robot Global Data.vi" "Solenoids"(w212) -> ()
      }
    }
    n129 = global write "Robot Global Data.vi" "Gyro Angle"(w184) -> ()
  }
  n130 = while {
    tunnel: w8 -> [w270]
    tunnel: w7 -> [w269]
    tunnel: w6 -> [w268]
    tunnel: w12 -> [w267]
    tunnel: w11 -> [w266]
    tunnel: w10 -> [w265]
    tunnel: w9 -> [w264]
    tunnel: w13 -> [w263]
    tunnel: w14 -> [w262]
    stop <- FALSE stop-if-true
    (unwired) "Front  Enter IR" ("refnum name")
    (unwired) "Rear Enter IR" ("refnum name")
    # "User wants Manual,\nand not in Autonomous"
    # "Load balls constantly when in auto"
    # "B10"
    # "Mag Roller"
    # "Rear Roller"
    # "Front Roller"
    # "B6"
    # "B8"
    # "B7"
    # "B5"
    # "B4"
    # "B2"
    # "B1"
    n131 = global read "Robot Global Data.vi" "RobotMode"() -> (w247:T1)
    n132 = Equal?(x=w247, y=WPI_DriverStationRobotMode."Autonomous Enabled" ("Robot Mode")) -> (x = y?=w227:bool)
    n133 = case shown="True" w227 {
      tunnel: [FALSE w273] -> w226
      frame False {
      }
      frame True {
        n134 = global read "Robot Global Data.vi" "Auto Load Balls State"() -> (w273:bool)
      }
    }
    n135 = Not(x=w227) -> (.not. x?=w230:bool)
    n136 = global read "Robot Global Data.vi" "Buttons"() -> (w251:T14)
    n137 = Unbundle By Name(w251) -> ("Button 1"=w249:bool, "Button 2"=w254:bool, "Button 4"=w250:bool, "Button 5"=w253:bool, "Button 6"=w257:bool, "Button 7"=w255:bool, "Button 8"=w256:bool, "Button 10"=w252:bool)  [unwired: 2 out]
    n138 = call "Button Toggle.vi"("Button Input"=w252) -> ("Toggled Output"=w232:bool)
    n139 = And(x=w232, y=w230) -> (x .and. y?=w231:bool)
    n140 = Not(x=w232) -> (.not. x?=w248:bool)
    n141 = global write "Robot Global Data.vi" "Automatic Mode"(w248) -> ()
    n142 = global read "Robot Global Data.vi" "Tracking"() -> (w236:bool)
    n143 = global read "Robot Global Data.vi" "RobotMode"() -> (w245:T1)
    n144 = Equal?(x=w245, y=WPI_DriverStationRobotMode."Autonomous Enabled" ("Robot Mode")) -> (x = y?=w235:bool)
    n145 = Or(x=w235, y=w236) -> (x .or. y?=w234:bool)
    n146 = global read "Robot Global Data.vi" "Shooter Controls"() -> (w233:T28)
    n147 = case shown="True" w234 {
      tunnel: w249 -> [w278 _]
      tunnel: [w278 w282] -> w243
      tunnel: w233 -> [w280 w281]
      tunnel: [w279 w281] -> w229
      frame False {
        # "update based on gamepad"
        n148 = Bundle By Name(cluster=w280, "Shooter Warmup"=w278) -> (w279:T28)
      }
      frame True {
        # "Use value provided by auto or tracking"
        n149 = Unbundle By Name(w281) -> ("Shooter Warmup"=w282:bool)
      }
    }
    n150 = case shown="False" w231 {
      tunnel: [w299 w815] -> w260
      tunnel: [w298 w814] -> w259
      tunnel: [w297 w813] -> w258
      tunnel: w267 -> [w342 _]
      tunnel: w266 -> [w341 _]
      tunnel: w265 -> [w340 _]
      tunnel: w264 -> [w339 _]
      tunnel: w243 -> [w288 w806]
      tunnel: w257 -> [w338 w808]
      tunnel: w256 -> [w337 w807]
      tunnel: w255 -> [w333 w809]
      tunnel: w253 -> [w332 w810]
      tunnel: w254 -> [w336 w811]
      tunnel: w250 -> [w335 w812]
      tunnel: [w334 w806] -> w242
      tunnel: w263 -> [w331 _]
      tunnel: w262 -> [w330 _]
      tunnel: w226 -> [w304 _]
      frame False {
        # "Drawback:\n - if a new ball found while another is \n     between IRs, it may lead to a jam"
        # "Ball finished"
        # "Once ball hasbeen processessed, enter \"Wait\""
        # "Enter IRs"
        # "Auto flag"
        # "Shoot"
        # "Changes: (7.16.12)\n - \"Stay in this case\" actually stays in the case\n - stopped rollers with ball run with Mag\n     (only when shooting clears a space for the ball)\n - if new ball found, update to next case"
        # "4"
        # "3"
        # "2"
        # "1"
        # "If Lower Mag AND [front/back] roller read, ignore Enter IR"
        # "Jam?"
        # "TODO: 4 balls, reverse rear roller\nCase 4, 8, 12: the rear mag can NEVER run. (or else, jam)"
        # "How many balls"
        # "B 1"
        # "B 6"
        # "B 8"
        # "B 7"
        # "B 5"
        # "B 4"
        # "B 2"
        # "B 1"
        # "Mag Roller"
        # "Rear Roller"
        # "Front Roller"
        # "1 - Front Roller IR\n2 - Back Roller IR\n3 - Lower Mag IR\n4 - Upper Mag IR"
        # "FWD"
        # "BKWD"
        # "FWD"
        # "BKWD"
        # "FWD"
        # "BKWD"
        # "FWD"
        n151 = call <vilib>:"WPI_DigitalInputGetValue.vi"("DigitalInputDevRef"=w342) -> ("Value"=w329:bool)  [unwired: 8 in, 2 out]
        n152 = call <vilib>:"WPI_DigitalInputGetValue.vi"("DigitalInputDevRef"=w341) -> ("Value"=w328:bool)  [unwired: 8 in, 2 out]
        n153 = call <vilib>:"WPI_DigitalInputGetValue.vi"("DigitalInputDevRef"=w340) -> ("Value"=w327:bool)  [unwired: 8 in, 2 out]
        n154 = call <vilib>:"WPI_DigitalInputGetValue.vi"("DigitalInputDevRef"=w339) -> ("Value"=w326:bool)  [unwired: 8 in, 2 out]
        n155 = call <vilib>:"WPI_DigitalInputGetValue.vi"("DigitalInputDevRef"=w330) -> ("Value"=w310:bool)  [unwired: 8 in, 2 out]
        n156 = call <vilib>:"WPI_DigitalInputGetValue.vi"("DigitalInputDevRef"=w331) -> ("Value"=w291:bool)  [unwired: 8 in, 2 out]
        n157 = Not(x=w310) -> (.not. x?=w311:bool)
        n158 = Not(x=w291) -> (.not. x?=w312:bool)
        n159 = Or(x=w311, y=w312) -> (x .or. y?=w306:bool)
        n160 = feedback #1() -> (w322:dbl)  [unwired: 1 in]
        n161 = global read "Robot Global Data.vi" "IR Values"() -> (w324:T29)
        n162 = Bundle By Name(cluster=w324, "Front Roller"=w329, "Back Roller"=w328, "Lower Mag"=w327, "Upper Mag"=w326, "Front Enter"=w310, "Rear Enter"=w291) -> (w325:T29)
        n163 = Build Array(w329, w328, w327, w326) -> (w344:bool[])
        n164 = Boolean Array To Number(Boolean array=w344) -> (number=w319:u32)
        n165 = Equal?(x=w319, y=u32 15) -> (x = y?=w320:bool)
        n166 = Select(t=w319, s=w320, f=w322) -> (s? t:f=w313:dbl)
        n167 = case shown="7" w313 {
          tunnel: [w787 w790 w801 1.0 ("f")] -> w323
          tunnel: w319 -> [w782 w791 w798 _]
          tunnel: [w775 w789 w795 FALSE] -> w317
          frame 15, Default {
            # "only wait for 7"
            # "Empty wait for ball"
            n168 = Equal?(x=u32 1, y=w782) -> (x = y?=w785:bool)
            n169 = Equal?(x=u32 3, y=w782) -> (x = y?=w784:bool)
            n170 = Or(x=w784, y=w785) -> (x .or. y?=w777:bool)
            n171 = Equal?(x=u32 7, y=w782) -> (x = y?=w783:bool)
            n172 = Or(x=w783, y=w777) -> (x .or. y?=w781:bool)
            n173 = call "Delayed Output.vi"("Interval (ms)"=u32 1000, "Input"=w781) -> ("Delayed Output"=w776:bool)
            n174 = Or(x=w777, y=w776) -> (x .or. y?=w775:bool)
            n175 = Select(t=w782, s=w775, f=15.0) -> (s? t:f=w787:dbl)
          }
          frame 7 {
            # "Ball in upper mag go to case 3 , stop rollers"
            n176 = Equal?(x=w791, y=u32 3) -> (x = y?=w789:bool)
            n177 = Select(t=3.0, s=w789, f=7.0) -> (s? t:f=w790:dbl)
          }
          frame 3 {
            # "2 balls go to case 1"
            n178 = Equal?(x=w798, y=2.0) -> (x = y?=w797:bool)
            n179 = Equal?(x=w798, y=u32 1) -> (x = y?=w796:bool)
            n180 = Or(x=w796, y=w797) -> (x .or. y?=w795:bool)
            n181 = Select(t=1.0, s=w795, f=3.0) -> (s? t:f=w801:dbl)
          }
          frame 1 {
            # "Full"
          }
        }
        n182 = feedback-in #1(w323) -> ()
        n183 = global write "Robot Global Data.vi" "IR Values"(w325) -> ()
        n184 = global read "Robot Global Data.vi" "Allow Fire"() -> (w343:bool)
        n185 = feedback #2(enum16{"Load Balls", "Shoot", "Wait"}."Wait") -> (w308:enum16{"Load Balls", "Shoot", "Wait"})
        n186 = Select(t=enum16{"Load Balls", "Shoot", "Wait"}."Wait", s=w317, f=w308) -> (s? t:f=w316:enum16{"Load Balls", "Shoot", "Wait"})
        n187 = Select(t=enum16{"Load Balls", "Shoot", "Wait"}."Load Balls", s=w306, f=w316) -> (s? t:f=w305:enum16{"Load Balls", "Shoot", "Wait"})
        n188 = Select(t=enum16{"Load Balls", "Shoot", "Wait"}."Load Balls", s=w304, f=w305) -> (s? t:f=w289:enum16{"Load Balls", "Shoot", "Wait"})
        n189 = Select(t=enum16{"Load Balls", "Shoot", "Wait"}."Load Balls", s=w288, f=w289) -> (s? t:f=w283:enum16{"Load Balls", "Shoot", "Wait"})
        n190 = global read "Robot Global Data.vi" "Ball State Machine"() -> (w286:T30)
        n191 = case shown="\"Load Balls\", Default" w283 {
          tunnel: [w381 0.0 ("Output") w762] -> w354
          tunnel: w343 -> [w378 _ w763]
          tunnel: w288 -> [w377 w749 w766]
          tunnel: [w376 w750 TRUE ("y")] -> w334
          tunnel: [w365 u32 0 u32 0] -> _
          tunnel: [w375 FALSE FALSE] -> _
          tunnel: [w374 TRUE FALSE] -> _
          tunnel: [w373 TRUE TRUE] -> _
          tunnel: w329 -> [w372 _ _]
          tunnel: w328 -> [w371 _ _]
          tunnel: w327 -> [w370 _ _]
          tunnel: w326 -> [w369 _ _]
          tunnel: w319 -> [w364 _ _]
          tunnel: [enum16{"Load Balls", "Shoot", "Wait"}."Load Balls" w760 w774] -> w318
          tunnel: [w368 w755 w762] -> w314
          tunnel: [w367 w755 w762] -> w315
          tunnel: w286 -> [w362 w747 w761]
          tunnel: [w361 w747 w761] -> w285
          frame "Load Balls", Default {
            # "State only updates when a\nNEW ball is read"
            n192 = feedback #3(u32 16) -> (w363:u32)
            n193 = case shown="1" w363 {
              selector: w363 -> [w393 w420 w447 w475 w499 w525 w551 w577 w589 w606 w622 w639 w656 w680 w706 _ _]
              tunnel: [w382 w413 w438 w476 w500 w526 w552 w578 1.0 ("Output") 1.0 ("Output") 1.0 ("Output") 1.0 ("Output") w668 w692 w716 w732 0.0 ("Output")] -> w381
              tunnel: w364 -> [w391 w410 w434 w464 w487 w510 w536 w565 w590 w603 w621 w638 w655 w679 w705 w731 w746]
              tunnel: [w392 w411 w436 w465 w488 w513 w539 w567 w591 w607 w623 w640 w657 w681 w704 w731 w746] -> w380
              tunnel: w372 -> [_ w409 _ w462 _ w512 _ w564 _ w605 _ w637 _ w678 _ _ _]
              tunnel: w371 -> [_ _ w435 w461 _ _ w538 w563 _ _ w620 w636 _ _ w702 _ _]
              tunnel: w370 -> [_ _ _ _ w486 w511 w537 w562 _ _ _ _ w654 w677 w701 _ _]
              tunnel: w369 -> [_ _ _ _ _ _ _ _ w588 w604 w619 w635 w653 w676 w700 _ _]
              tunnel: [w390 w419 w446 w474 w498 w524 w550 w576 w600 w616 w632 w650 w667 w691 w715 w730 FALSE ("y")] -> w376
              tunnel: w378 -> [w389 w418 w445 w473 w497 w523 w549 w575 _ _ _ _ w666 w690 w703 w729 _]
              tunnel: w377 -> [w388 w417 w444 w472 w496 w522 w548 w574 w599 w615 w631 w649 w665 w689 w714 w728 _]
              tunnel: [u32 4 u32 3 u32 3 u32 2 u32 3 u32 2 u32 2 u32 1 u32 3 u32 2 u32 2 u32 1 u32 2 u32 1 u32 1 u32 0 u32 0] -> w365
              tunnel: [FALSE w415 FALSE FALSE FALSE TRUE FALSE w572 FALSE TRUE FALSE w646 FALSE TRUE FALSE w726 w742] -> w374
              tunnel: [w385 FALSE w441 FALSE TRUE FALSE TRUE w572 TRUE FALSE TRUE w646 TRUE FALSE TRUE w726 w742] -> w373
              tunnel: [FALSE FALSE FALSE FALSE TRUE FALSE FALSE FALSE TRUE FALSE FALSE FALSE TRUE FALSE FALSE FALSE FALSE] -> w375
              tunnel: [-1.0 ("Output") w413 0.0 ("Output") w467 0.0 ("Output") 1.0 ("Output") 1.0 ("Output") w570 0.0 ("Output") w609 w625 1.0 ("Output") 0.0 ("Output") w684 w709 w724 w740] -> w368
              tunnel: [w382 0.0 ("Output") w438 w467 1.0 ("Output") 1.0 ("Output") 1.0 ("Output") w570 1.0 ("Output") w609 w625 1.0 ("Output") 1.0 ("Output") w684 w709 w724 w740] -> w367
              frame 0, Default {
                # "front roller\nrun w/ Mag"
                # "reverse\nrear roller"
                # "FFFF 4 Balls"
                n194 = case shown="True" w388 {
                  tunnel: [0.0 ("Output") w400] -> w382
                  tunnel: w393 -> [_ w398]
                  tunnel: [w397 w398] -> w392
                  tunnel: w391 -> [w397 _]
                  tunnel: [FALSE TRUE] -> w390
                  tunnel: w389 -> [_ w401]
                  tunnel: [FALSE w399] -> w385
                  frame False {
                    # "Continue to next case"
                  }
                  frame True {
                    # "Stay in this case"
                    n195 = case shown="True" w401 {
                      tunnel: [0.0 ("Output") 1.0 ("Output")] -> w400
                      tunnel: [FALSE TRUE] -> w399
                      frame False {
                      }
                      frame True {
                      }
                    }
                  }
                }
              }
              frame 1 {
                # "rear roller\nrun w/ Mag"
                # "new ball in front,\nupdate state"
                # "Full"
                # "TFFF No ball in front roller"
                n196 = case shown="True" w417 {
                  tunnel: [0.0 ("Output") w427] -> w413
                  tunnel: w410 -> [w423 _]
                  tunnel: [w423 w425] -> w412
                  tunnel: w420 -> [_ w425]
                  tunnel: [FALSE TRUE] -> w419
                  tunnel: w418 -> [_ w428]
                  tunnel: [FALSE w426] -> w415
                  frame False {
                    # "Continue to next case"
                    # "Wait for button 4"
                  }
                  frame True {
                    # "Stay in this case"
                    # "Shoot balls :)"
                    n197 = case shown="True" w428 {
                      tunnel: [0.0 ("Output") 1.0 ("Output")] -> w427
                      tunnel: [FALSE TRUE] -> w426
                      frame False {
                      }
                      frame True {
                      }
                    }
                  }
                }
                n198 = Select(t=w412, s=w409, f=w410) -> (s? t:f=w411:u32)
              }
              frame 2 {
                # "new ball in rear,\nupdate state"
                # "front roller\nrun w/ Mag"
                # "Full"
                # "FTFF Rear roller no ball"
                n199 = case shown="True" w444 {
                  tunnel: [0.0 ("Output") w454] -> w438
                  tunnel: [w450 w452] -> w437
                  tunnel: w434 -> [w450 _]
                  tunnel: w447 -> [_ w452]
                  tunnel: [FALSE TRUE ("y")] -> w446
                  tunnel: w445 -> [_ w455]
                  tunnel: [FALSE w453] -> w441
                  frame False {
                    # "Continue to next case"
                    # "Wait for button 4"
                  }
                  frame True {
                    # "Stay in this case"
                    # "Shoot balls :)"
                    n200 = case shown="True" w455 {
                      tunnel: [0.0 ("Output") 1.0 ("Output")] -> w454
                      tunnel: [FALSE TRUE] -> w453
                      frame False {
                      }
                      frame True {
                      }
                    }
                  }
                }
                n201 = Select(t=w437, s=w435, f=w434) -> (s? t:f=w436:u32)
              }
              frame 3 {
                w467 = 1.0 ("Output")
                # "new ball in either roller,\nupdate state"
                # "TTFF 2 Balls in magazine"
                n202 = case shown="True" w472 {
                  tunnel: [0.0 ("Output") w483] -> w476
                  tunnel: [w478 w480] -> w466
                  tunnel: w475 -> [_ w480]
                  tunnel: w464 -> [w478 _]
                  tunnel: [FALSE ("y") TRUE ("y")] -> w474
                  tunnel: w473 -> [_ w481]
                  frame False {
                    # "Continue to next case"
                    # "Rollers run while button\nnot pressed"
                  }
                  frame True {
                    # "Stay in this case"
                    # "Fire when button is pressed"
                    n203 = case shown="True" w481 {
                      tunnel: [0.0 ("Output") 1.0 ("Output")] -> w483
                      frame False {
                      }
                      frame True {
                      }
                    }
                  }
                }
                n204 = And(x=w462, y=w461) -> (x .and. y?=w463:bool)
                n205 = Select(t=w466, s=w463, f=w464) -> (s? t:f=w465:u32)
              }
              frame 4 {
                # "new ball in lower Mag,\nupdate state"
                # "NOT w/ Mag"
                # "!!JAM!!"
                # "FFTF Balls in both rollers, and upper mag"
                n206 = case shown="True" w496 {
                  tunnel: [0.0 ("Output") w507] -> w500
                  tunnel: [w502 w504] -> w489
                  tunnel: w499 -> [_ w504]
                  tunnel: w487 -> [w502 _]
                  tunnel: [FALSE ("y") TRUE ("y")] -> w498
                  tunnel: w497 -> [_ w505]
                  frame False {
                    # "Continue to next case"
                    # "Only run front roller"
                  }
                  frame True {
                    # "Stay in this case"
                    # "Fire and load from front"
                    n207 = case shown="True" w505 {
                      tunnel: [0.0 ("Output") 1.0 ("Output")] -> w507
                      frame False {
                      }
                      frame True {
                      }
                    }
                  }
                }
                n208 = Select(t=w489, s=w486, f=w487) -> (s? t:f=w488:u32)
              }
              frame 5 {
                # "new ball in front or\nlower Mag, update state"
                # "TFTF Ball in Upper Mag, and Rear Roller"
                n209 = case shown="True" w522 {
                  tunnel: [0.0 ("Output") w533] -> w526
                  tunnel: w510 -> [w528 _]
                  tunnel: [w528 w530] -> w514
                  tunnel: w525 -> [_ w530]
                  tunnel: [FALSE ("y") TRUE ("y")] -> w524
                  tunnel: w523 -> [_ w531]
                  frame False {
                    # "Continue to next case"
                    # "Load rollers"
                  }
                  frame True {
                    # "Stay in this case"
                    # "Fire and load"
                    n210 = case shown="True" w531 {
                      tunnel: [0.0 ("Output") 1.0 ("Output")] -> w533
                      frame False {
                      }
                      frame True {
                      }
                    }
                  }
                }
                n211 = And(x=w512, y=w511) -> (x .and. y?=w515:bool)
                n212 = Select(t=w514, s=w515, f=w510) -> (s? t:f=w513:u32)
              }
              frame 6 {
                # "new ball in rear or\nlower Mag, update state"
                # "FTTF Ball in front roller and top mag"
                n213 = case shown="False" w548 {
                  tunnel: [0.0 ("Output") w559] -> w552
                  tunnel: [w554 w556] -> w540
                  tunnel: w551 -> [_ w556]
                  tunnel: w536 -> [w554 _]
                  tunnel: [FALSE ("y") TRUE ("y")] -> w550
                  tunnel: w549 -> [_ w557]
                  frame False {
                    # "Continue to next case"
                    # "Load balls"
                  }
                  frame True {
                    # "Stay in this case"
                    # "Fire and load"
                    n214 = case shown="True" w557 {
                      tunnel: [0.0 ("Output") 1.0 ("Output")] -> w559
                      frame False {
                      }
                      frame True {
                      }
                    }
                  }
                }
                n215 = And(x=w538, y=w537) -> (x .and. y?=w541:bool)
                n216 = Select(t=w540, s=w541, f=w536) -> (s? t:f=w539:u32)
              }
              frame 7 {
                w570 = 1.0 ("Output")
                w572 = FALSE
                # "new ball in any,\nupdate state"
                # "TTTF Ball in upper mag"
                n217 = case shown="True" w574 {
                  tunnel: [0.0 ("Output") w585] -> w578
                  tunnel: [w580 w582] -> w568
                  tunnel: w577 -> [_ w582]
                  tunnel: w565 -> [w580 _]
                  tunnel: [FALSE ("y") TRUE ("y")] -> w576
                  tunnel: w575 -> [_ w583]
                  frame False {
                    # "Continue to\nnext case"
                    # "Load balls"
                  }
                  frame True {
                    # "Stay in this case"
                    # "Fire and load"
                    n218 = case shown="False" w583 {
                      tunnel: [0.0 ("Output") 1.0 ("Output")] -> w585
                      frame False {
                      }
                      frame True {
                      }
                    }
                  }
                }
                n219 = And(x=w563, y=w562) -> (x .and. y?=w566:bool)
                n220 = And(x=w564, y=w566) -> (x .and. y?=w569:bool)
                n221 = Select(t=w568, s=w569, f=w565) -> (s? t:f=w567:u32)
              }
              frame 8 {
                # "new ball in upper Mag,\nupdate state"
                # "!!JAM!!"
                # "Run front roller\nand magazine"
                # "FFFT Balls in front, rear, and lower mag"
                n222 = case shown="True" w599 {
                  tunnel: [FALSE ("y") TRUE ("y")] -> w600
                  frame False {
                  }
                  frame True {
                  }
                }
                n223 = Select(t=w589, s=w588, f=w590) -> (s? t:f=w591:u32)
              }
              frame 9 {
                w609 = 1.0 ("Output")
                # "new ball in front or upper Mag,\nupdate state"
                # "Load balls to top"
                # "TFFT Ball in rear loader, and lower mag"
                n224 = case shown="True" w615 {
                  tunnel: [FALSE ("y") TRUE ("y")] -> w616
                  frame False {
                  }
                  frame True {
                  }
                }
                n225 = And(x=w605, y=w604) -> (x .and. y?=w608:bool)
                n226 = Select(t=w606, s=w608, f=w603) -> (s? t:f=w607:u32)
              }
              frame 10 {
                w625 = 1.0 ("Output")
                # "new ball in rear or upper Mag,\nupdate state"
                # "FTFT Ball in front and lower mag"
                n227 = case shown="True" w631 {
                  tunnel: [FALSE ("y") TRUE ("y")] -> w632
                  frame False {
                  }
                  frame True {
                  }
                }
                n228 = And(x=w620, y=w619) -> (x .and. y?=w624:bool)
                n229 = Select(t=w622, s=w624, f=w621) -> (s? t:f=w623:u32)
              }
              frame 11 {
                w646 = FALSE
                # "new ball in any,\nupdate state"
                # "TTFT Ball in lower mag"
                n230 = case shown="True" w649 {
                  tunnel: [FALSE ("y") TRUE ("y")] -> w650
                  frame False {
                  }
                  frame True {
                  }
                }
                n231 = And(x=w636, y=w635) -> (x .and. y?=w641:bool)
                n232 = And(x=w637, y=w641) -> (x .and. y?=w642:bool)
                n233 = Select(t=w639, s=w642, f=w638) -> (s? t:f=w640:u32)
              }
              frame 12 {
                # "new ball in Mag,\nupdate state"
                # "!!JAM!!"
                # "Load front ball to mag"
                # "FFTT Balls in front and back roller"
                n234 = case shown="True" w665 {
                  tunnel: [0.0 ("Output") w672] -> w668
                  tunnel: [FALSE ("y") TRUE ("y")] -> w667
                  tunnel: w666 -> [_ w671]
                  frame False {
                  }
                  frame True {
                    n235 = case shown="False" w671 {
                      tunnel: [0.0 ("Output") 1.0 ("Output")] -> w672
                      frame False {
                      }
                      frame True {
                      }
                    }
                  }
                }
                n236 = And(x=w654, y=w653) -> (x .and. y?=w658:bool)
                n237 = Select(t=w656, s=w658, f=w655) -> (s? t:f=w657:u32)
              }
              frame 13 {
                w684 = 1.0 ("Output")
                # "new ball in any,\nupdate state"
                # "Load rear ball\n(run front roller)"
                # "TFTT Ball in rear roller"
                n238 = case shown="True" w689 {
                  tunnel: [0.0 ("Output") w696] -> w692
                  tunnel: [FALSE ("y") TRUE ("y")] -> w691
                  tunnel: w690 -> [_ w695]
                  frame False {
                  }
                  frame True {
                    n239 = case shown="True" w695 {
                      tunnel: [0.0 ("Output") 1.0 ("Output")] -> w696
                      frame False {
                      }
                      frame True {
                      }
                    }
                  }
                }
                n240 = And(x=w677, y=w676) -> (x .and. y?=w682:bool)
                n241 = And(x=w678, y=w682) -> (x .and. y?=w683:bool)
                n242 = Select(t=w680, s=w683, f=w679) -> (s? t:f=w681:u32)
              }
              frame 14 {
                w709 = 1.0 ("Output")
                # "Load front ball\n(run rear roller)"
                # "FTTT Ball in front roller"
                n243 = case shown="True" w714 {
                  tunnel: [0.0 ("t") w721] -> w716
                  tunnel: [FALSE ("y") TRUE ("y")] -> w715
                  tunnel: w703 -> [_ w719]
                  frame False {
                  }
                  frame True {
                    n244 = case shown="True" w719 {
                      tunnel: [0.0 ("Output") 1.0 ("Output")] -> w721
                      frame False {
                      }
                      frame True {
                      }
                    }
                  }
                }
                n245 = And(x=w701, y=w700) -> (x .and. y?=w707:bool)
                n246 = And(x=w702, y=w707) -> (x .and. y?=w708:bool)
                n247 = Select(t=w706, s=w708, f=w705) -> (s? t:f=w704:u32)
              }
              frame 15 {
                w724 = 1.0 ("Output")
                w726 = FALSE
                # "Run both rollers"
                # "1"
                # "2"
                # "3"
                # "4"
                # "TTTT No balls"
                n248 = case shown="True" w728 {
                  tunnel: [0.0 ("Output") w736] -> w732
                  tunnel: [FALSE ("y") TRUE ("y")] -> w730
                  tunnel: w729 -> [_ w735]
                  frame False {
                  }
                  frame True {
                    n249 = case shown="True" w735 {
                      tunnel: [0.0 ("Output") 1.0 ("Output")] -> w736
                      frame False {
                      }
                      frame True {
                      }
                    }
                  }
                }
              }
              frame 16 {
                w740 = 0.0 ("Output")
                w742 = FALSE
                # "When the loop starts (default case)"
              }
            }
            n250 = feedback-in #3(w380) -> ()
            n251 = Bundle By Name(cluster=w362, "Current State"=w363, "Reading State"=w364, "Number of Balls"=w365) -> (w361:T30)
          }
          frame "Wait" {
            w755 = 0.0 ("Output")
            n252 = Select(t=enum16{"Load Balls", "Shoot", "Wait"}."Load Balls", s=w749, f=enum16{"Load Balls", "Shoot", "Wait"}."Wait") -> (s? t:f=w760:enum16{"Load Balls", "Shoot", "Wait"})
            n253 = Select(t=TRUE ("y"), s=w749, f=FALSE ("y")) -> (s? t:f=w750:bool)
          }
          frame "Shoot" {
            # "NOTE:"
            # "This state is DISABLED:\nAll shooting should be done in \"Load Balls\"\nbecause the 0-15 states should determine\nthe reaction of each roller on the Allow Fire\nflag."
            # "Stop all rollers until Allow Fire is true"
            n254 = Select(t=1.0 ("Output"), s=w763, f=0.0 ("Output")) -> (s? t:f=w762:dbl)
            n255 = Select(t=enum16{"Load Balls", "Shoot", "Wait"}."Load Balls", s=w766, f=enum16{"Load Balls", "Shoot", "Wait"}."Wait") -> (s? t:f=w774:enum16{"Load Balls", "Shoot", "Wait"})
          }
        }
        n256 = feedback-in #2(w318) -> ()
        n257 = Bundle By Name(cluster=w285, "State"=w283) -> (w284:T30)
        n258 = global write "Robot Global Data.vi" "Ball State Machine"(w284) -> ()
        n259 = Select(t=-1.0, s=w336, f=w354) -> (s? t:f=w351:dbl)
        n260 = Select(t=1.0, s=w335, f=w351) -> (s? t:f=w300:dbl)
        n261 = Select(t=-1.0, s=w333, f=w314) -> (s? t:f=w348:dbl)
        n262 = Select(t=1.0, s=w332, f=w348) -> (s? t:f=w301:dbl)
        n263 = global read "Robot Global Data.vi" "RobotMode"() -> (w294:T1)
        n264 = Select(t=-1.0, s=w337, f=w315) -> (s? t:f=w347:dbl)
        n265 = global read "Robot Global Data.vi" "Feed Balls"() -> (w295:bool)
        n266 = Select(t=1.0, s=w338, f=w347) -> (s? t:f=w302:dbl)
        n267 = Equal?(x=w294, y=WPI_DriverStationRobotMode."Autonomous Enabled" ("Robot Mode")) -> (x = y?=w292:bool)
        n268 = And(x=w295, y=w292) -> (x .and. y?=w296:bool)
        n269 = case shown="True" w296 {
          tunnel: w302 -> [w357 _]
          tunnel: w301 -> [w356 _]
          tunnel: w300 -> [w355 _]
          tunnel: [w357 -1.0 ("Output")] -> w299
          tunnel: [w356 -1.0 ("Output")] -> w298
          tunnel: [w355 0.0 ("Output")] -> w297
          frame False {
            # "No\nchanges"
          }
          frame True {
            # "Mag\nstopped"
            # "Both\nramps\nback-\nwards"
          }
        }
      }
      frame True {
        n270 = case shown="False" w808 {
          tunnel: [w827 1.0 ("y")] -> w815
          tunnel: w807 -> [w826 _]
          frame False {
            n271 = case shown="True" w826 {
              tunnel: [0.0 ("y") -1.0 ("y")] -> w827
              frame False {
              }
              frame True {
              }
            }
          }
          frame True {
          }
        }
        n272 = case shown="False" w812 {
          tunnel: [w817 1.0 ("y")] -> w813
          tunnel: w811 -> [w816 _]
          frame False {
            n273 = case shown="True" w816 {
              tunnel: [0.0 ("y") -1.0 ("y")] -> w817
              frame False {
              }
              frame True {
              }
            }
          }
          frame True {
          }
        }
        n274 = case shown="False" w810 {
          tunnel: [w822 1.0 ("y")] -> w814
          tunnel: w809 -> [w821 _]
          frame False {
            n275 = case shown="True" w821 {
              tunnel: [0.0 ("y") -1.0 ("y")] -> w822
              frame False {
              }
              frame True {
              }
            }
          }
          frame True {
          }
        }
      }
    }
    n276 = call <vilib>:"WPI_MotorControlSetOutput.vi"("Output"=w260, "MotorControlDevRef"=w270) -> ()  [unwired: 8 in, 2 out]
    n277 = call <vilib>:"WPI_MotorControlSetOutput.vi"("Output"=w259, "MotorControlDevRef"=w269) -> ()  [unwired: 8 in, 2 out]
    n278 = call <vilib>:"WPI_MotorControlSetOutput.vi"("Output"=w258, "MotorControlDevRef"=w268) -> ()  [unwired: 8 in, 2 out]
    n279 = global read "Robot Global Data.vi" "RobotMode"() -> (w241:T1)
    n280 = Wait (ms)(milliseconds to wait=u32 50) -> ()  [unwired: 1 out]
    n281 = global read "Robot Global Data.vi" "Tracking"() -> (w237:bool)
    n282 = Equal?(x=w241, y=WPI_DriverStationRobotMode."Autonomous Enabled" ("Robot Mode")) -> (x = y?=w239:bool)
    n283 = Or(x=w237, y=w239) -> (x .or. y?=w238:bool)
    n284 = case shown="True" w238 {
      tunnel: w242 -> [w276 _]
      tunnel: w229 -> [w275 w277]
      tunnel: [w274 w277] -> w228
      frame False {
        n285 = Bundle By Name(cluster=w275, "Shooter Warmup"=w276) -> (w274:T28)
      }
      frame True {
        # "Autonomous\n(or tracking)\nhas control\nof shooter"
      }
    }
    n286 = global write "Robot Global Data.vi" "Shooter Controls"(w228) -> ()
  }
  n287 = while {
    stop <- FALSE stop-if-true
    # "This global is written to in the Autonomous and Teleop VIs"
    # "Flash the USER1 LED with the rate controlled from Autonomous and Teleop"
    n288 = global read "Robot Global Data.vi" "LED toggle rate (ms)"() -> (w831:u32)
    n289 = call <vilib>:"WPI_UtilitiesFRC LEDs.vi"("State"=FPGA_UtilitiesLED_State."Toggle", "LED Type"=FPGA_UtilitiesLED_Source."User LED") -> ()  [unwired: 1 in, 9 out]
    n290 = Wait (ms)(milliseconds to wait=w831) -> ()  [unwired: 1 out]
  }
